vi "Load Data.vi"(2 "error in (no error)":errorcluster, 3 "History Data":T1) -> (0 "error out":errorcluster, 1 "History Data Output":T1)   [LabVIEW 2021]
doc: "Este VI lee los datos de un fichero datalog con el formato indicado con el cluster de entrada"
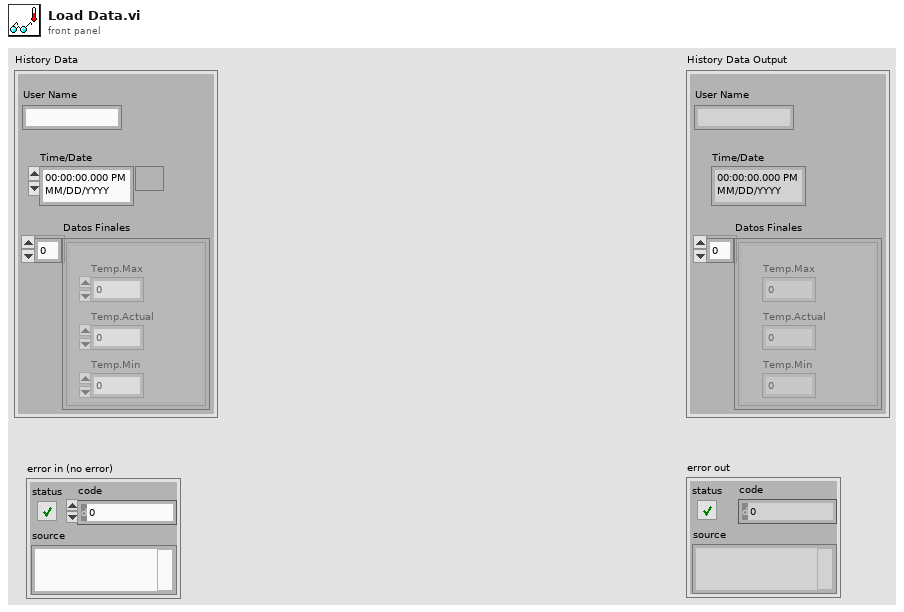
[diagram p1: front panel]
types:
  T1 = cluster{"User Name":string, "Time/Date":timestamp, "Datos Finales":cluster{"Temp.Max":dbl, "Temp.Actual":dbl, "Temp.Min":dbl}[]}
  T2 = cluster{"Temp.Max":dbl, "Temp.Actual":dbl, "Temp.Min":dbl}[]
  T3 = enum16{"open", "replace", "create", "open or create", "replace or create", "replace or create with confirmation"}
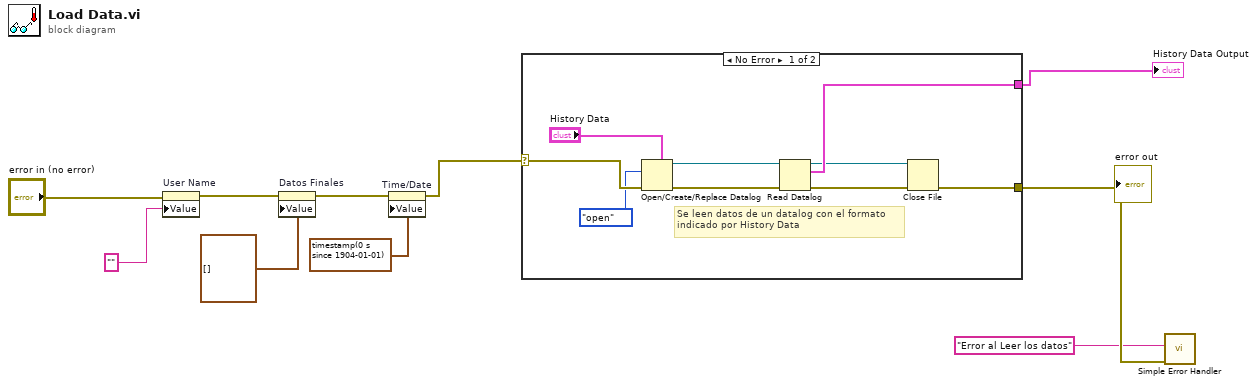
[diagram p0: block diagram]
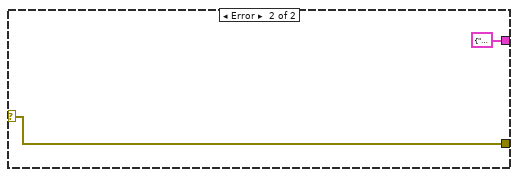
[diagram p2: hidden frame]
diagram:
  n1 = property on="User Name" class="Str"(error in="error in (no error)", "Value"="") -> (error out=w9:errorcluster)  [unwired: 1 in, 1 out]
  n2 = property on="Datos Finales" class="Arr (strict)"(error in=w9, "Value"=T2 []) -> (error out=w8:errorcluster)  [unwired: 1 in, 1 out]
  n3 = property on="Time/Date" class="AbsTime (strict)"(error in=w8, "Value"=timestamp(0 s since 1904-01-01)) -> (error out=w4:errorcluster)  [unwired: 1 in, 1 out]
  n4 = case shown="No Error" w4 {
    selector: w4 -> [w18 w21]
    tunnel: [w17 w21] -> w3
    tunnel: [w13 T1 {"User Name"="", "Time/Date"=timestamp(0 s since 1904-01-01), "Datos Finales"=[]} ("History Data")] -> w1
    frame No Error {
      # "Se leen datos de un datalog con el formato\nindicado por History Data"
      n5 = Open/Create/Replace Datalog(5:"History Data", 8:w18, 10:T3."open" ("operation (0:open)")) -> (0:w15:errorcluster, 3:w16:refnum<k1>)  [unwired: 3 in, 1 out]
      n6 = Read Datalog(4:w15, 7:w16) -> (0:w14:errorcluster, 2:w13:T1, 3:w12:refnum<k1>)  [unwired: 1 in]
      n7 = Close File(refnum=w12, error in=w14) -> (error out=w17:errorcluster)  [unwired: 1 out]
    }
    frame Error {
    }
  }
  "error out" <- w3
  "History Data Output" <- w1
  n8 = call <vilib>:"Simple Error Handler.vi"("error source (\" \")"="Error al Leer los datos" ("error source (\" \")"), "error in (no error)"=w3) -> ()  [unwired: 3 in, 5 out]
